vi "myRIO testing.vi"() -> (0 "Accelerometer":cluster{"Z":i16, "Y":i16, "X":i16} {"X" scale=-300.0..300.0; "Y" scale=-300.0..300.0; "Z" scale=-300.0..300.0})   [LabVIEW 2015, in "Everything.lvlib"]
uses:
  Everything.lvlib
  <vilib>/userdefined/High Color/IMAQdx.ctl
  <vilib>/myRIO/Common/Instrument Driver Framework/myRIO v1.0/UART/vis/myRIO v1.0 Close UART.vi
  <vilib>/FPGAPlugInAG/myRIO-1900/niLvFpga_Open_myRIO-1900.vi
  <vilib>/rvi/interface/common/dynamic/niFpgaDynamicAddResources.vi
  <vilib>/FPGAPlugInAG/Dynamic/niLvFpga_Run_Dynamic.vi
  <vilib>/Utility/error.llb/Error Cluster From Error Code.vi
  <vilib>/rvi/errors/niLvFpgaAdjustHostInterfaceError.vi
  <vilib>/FPGAPlugInAG/Dynamic/niLvFpga_Close_Dynamic.vi
  <vilib>/myRIO/Common/Instrument Driver Framework/Utilities/vis/FPGA Ref Manager.vi
  <vilib>/myRIO/Common/Instrument Driver Framework/myRIO v1.0/myRIO v1.0 Reset FPGA.vi
  <vilib>/myRIO/Common/Instrument Driver Framework/myRIO v1.0/IRQ/vis/myRIO v1.0 IRQ Info FGV.vi
  <vilib>/myRIO/Common/Instrument Driver Framework/myRIO v1.0/IRQ/vis/myRIO v1.0 Timer IRQ Info FGV.vi
  <vilib>/myRIO/Common/Instrument Driver Framework/myRIO v1.0/IRQ/vis/myRIO v1.0 ISR Agent.vi
  <vilib>/rvi/interface/nirviOpenFPGA/nirviOpenFPGA.xnode
  FPGA Bitfiles/PDMSMain_FPGATarget-Wi-Fi_Express2_Jo8xc+hAvHc.lvbitx
  FPGA/Express.vi
  <vilib>/rvi/interface/nirviMethod/nirviMethod.xnode
  <vilib>/rvi/interface/nirviReadWriteControl/nirviReadWriteControl.xnode
  <vilib>/rvi/interface/nirviCloseFPGA/nirviCloseFPGA.xnode
  <vilib>/myRIO/Instrument Drivers/Utilities/Utilities.lvlib
  NiFpgaLv.dll
  <vilib>/rvi/interface/Simulation/niFpgaSimulationCallBeginRW.vi
panel:
  in  "LED 0":T1 {"Brightness" max=1000}
  in  "LED 2":T2 {"Brightness" max=1000}
  in  "LED 1":T3 {"Brightness" max=1000}
  in  "LED 3":T4 {"Brightness" max=1000}
  out "IR":cluster{"1":bool, "2":bool}
  out "Image":T5(plugin-control)
  out "Error Out":errorcluster
  in  "Mot F":T6
  out "Button":bool
  out "PIR":bool
  in  "Stop Button":bool
  out "BOOL O/P":T7
  out "CM O/P":cluster{"US BK":u32, "US FL":u32, "US FR":u32}
  # "Obstacle"
  # "Robot's Position"
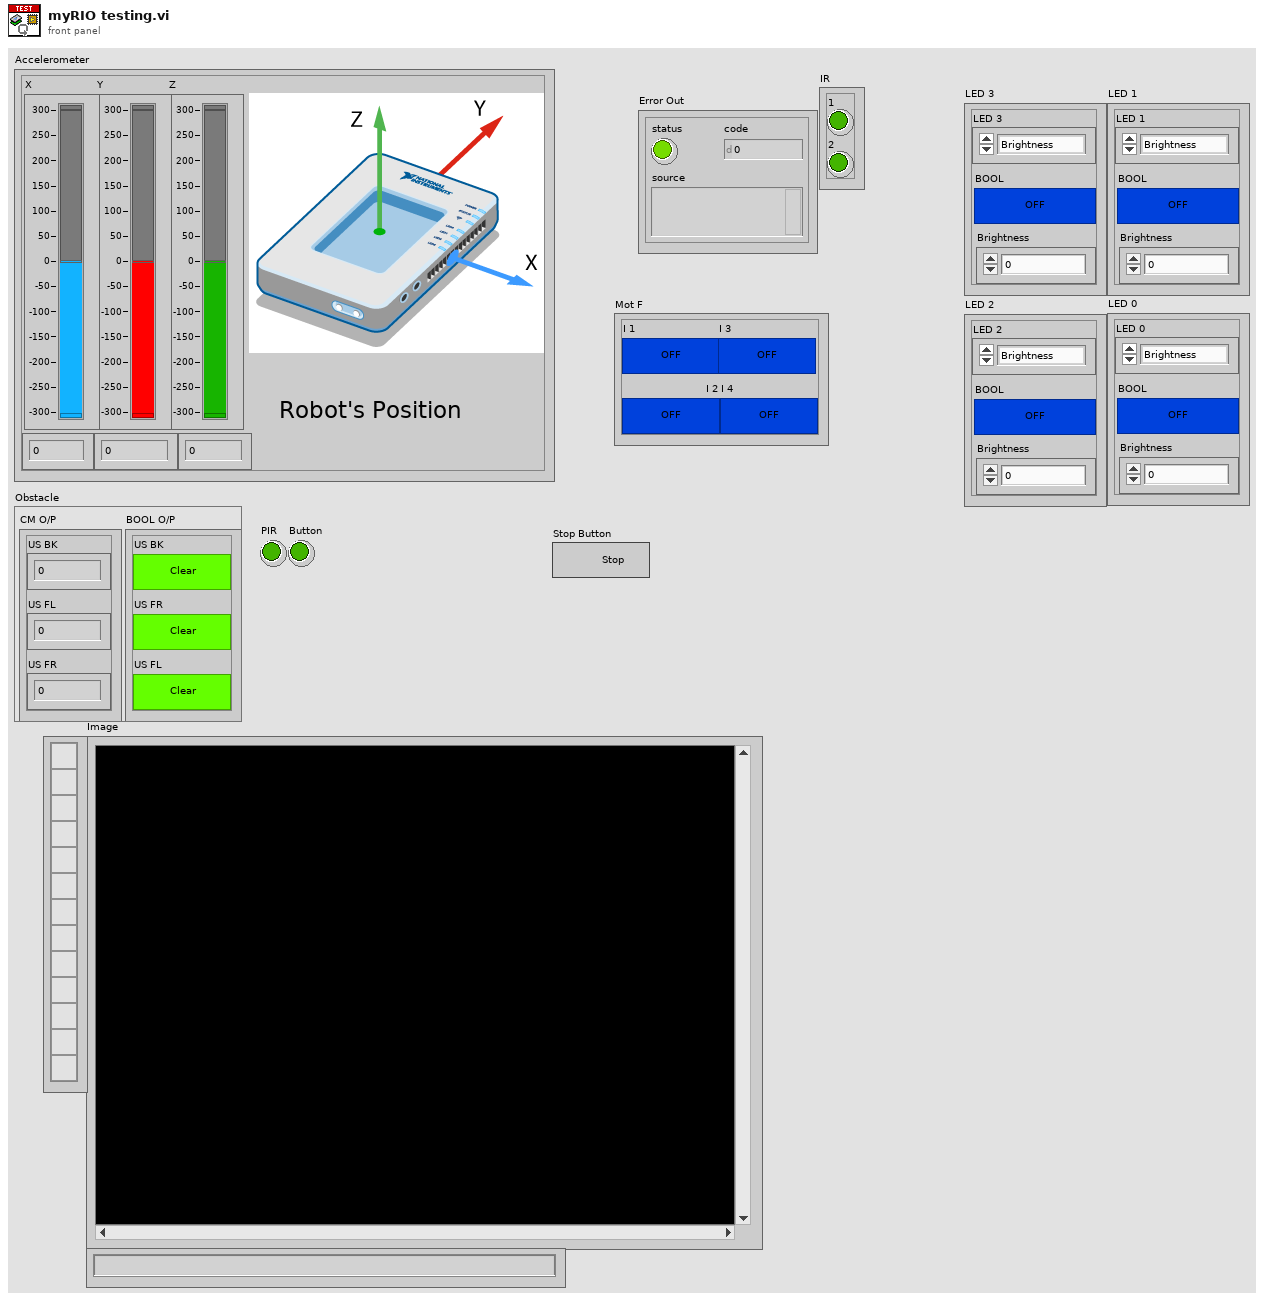
[diagram p1: front panel]
types:
  T1 = cluster{"LED 0":enum16{"Brightness", "Bool"}, "BOOL":bool, "Brightness":u32}
  T2 = cluster{"LED 2":enum16{"Brightness", "Bool"}, "BOOL":bool, "Brightness":u32}
  T3 = cluster{"LED 1":enum16{"Brightness", "Bool"}, "BOOL":bool, "Brightness":u32}
  T4 = cluster{"LED 3":enum16{"Brightness", "Bool"}, "BOOL":bool, "Brightness":u32}
  T5 = typedef "IMAQ Image.ctl" = refnum<image>
  T6 = cluster{"I 1":bool, "I 2":bool, "I 3":bool, "I 4":bool}
  T7 = cluster{"US BK":bool, "US FR":bool, "US FL":bool}
  T8 = typedef "IMAQdx.ctl" = refnum<k21>
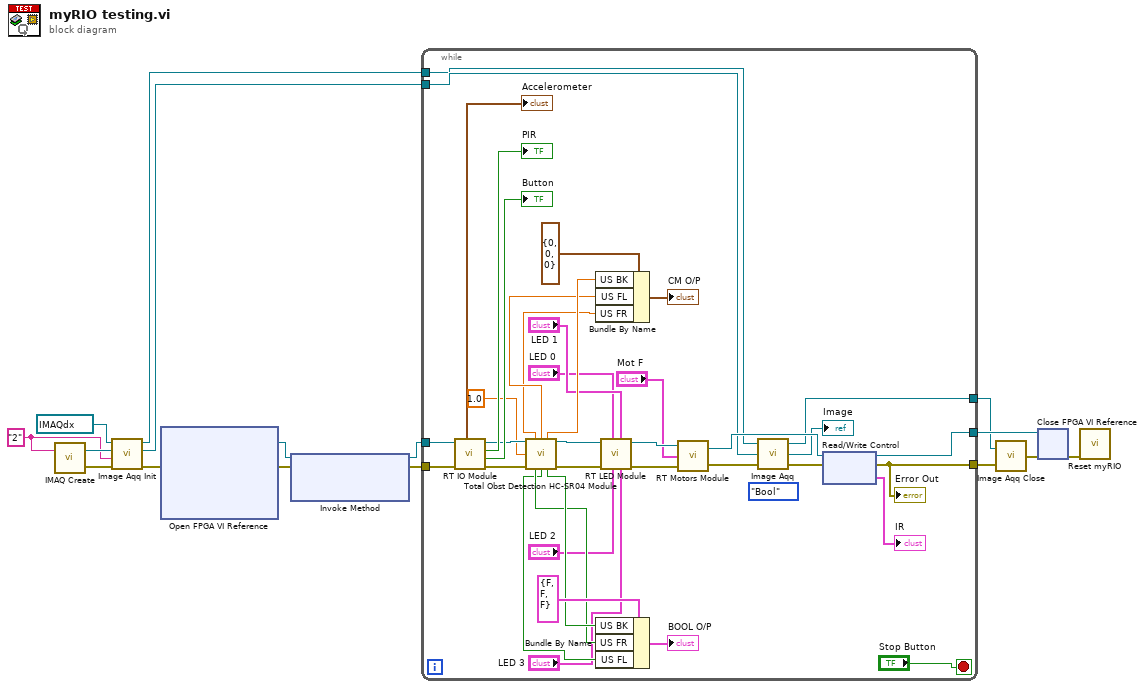
[diagram p0: block diagram]
diagram:
  w8 = "2" ("Image Name")
  n1 = call "IMAQ Create"("Image Name"=w8) -> ("New Image"=w14:T5, "error out"=w9:errorcluster)  [unwired: 4 in]
  n2 = call "Image Aqq Init.vi"("Error In"=w9, "Img Name In"=w8, "Img In"=w14, "Camera"=T8 "cam0") -> ("Error Out"=w7:errorcluster, "Img Out"=w12:T5, "Cam Out"=w11:T8)  [unwired: 1 out]
  n3 = xnode "Open FPGA VI Reference"("error in"=w7) -> ("FPGA VI Reference Out"=w4:refnum<k20>, "error out"=w3:errorcluster)  [unwired: 1 in]
  n4 = xnode "Invoke Method"("FPGA VI Reference In"=w4, "error in"=w3) -> ("FPGA VI Reference Out"=w2:refnum<k20>, "error out"=w1:errorcluster)  [unwired: 1 in]
  n5 = while {
    tunnel: w1 -> [w54]
    tunnel: [w34] -> w16
    tunnel: w2 -> [w32]
    tunnel: [w29] -> w13
    tunnel: w12 -> [w26]
    tunnel: w11 -> [w25]
    tunnel: [w24] -> w10
    stop <- "Stop Button" stop-if-true
    (unwired) enum16{"Brightness", "Bool"}."Bool" ("LED")
    n6 = call "RT IO Module.vi"("FPGA VI Reference In"=w32, "Error In"=w54) -> ("Accelerometer"=→"Accelerometer":cluster{"Z":i16, "Y":i16, "X":i16}, "FPGA VI Reference Out"=w31:refnum<k20>, "PIR"=→"PIR":bool, "Button"=→"Button":bool, "Error Out"=w51:errorcluster)  [unwired: 2 in, 2 out]
    n7 = call "Total Obst Detection HC-SR04 Module.vi"("FPGA VI Reference In"=w31, "Threshold"=sgl 1.0, "Error In"=w51) -> (1:"US FR"=w44:sgl, 2:"US FL"=w45:sgl, 3:"US BK"=w46:sgl, "FPGA VI Reference Out"=w39:refnum<k20>, 12:"US FR"=w42:bool, 13:"US FL"=w41:bool, 14:"US BK"=w43:bool, "Error Out"=w40:errorcluster)  [unwired: 5 in]
    n8 = Bundle By Name(cluster=cluster{"US BK":u32, "US FL":u32, "US FR":u32} {"US BK"=0, "US FL"=0, "US FR"=0} ("CM O/P 2"), "US BK"=w46, "US FL"=w45, "US FR"=w44) -> (→"CM O/P":cluster{"US BK":u32, "US FL":u32, "US FR":u32})
    n9 = Bundle By Name(cluster=T7 {"US BK"=FALSE, "US FR"=FALSE, "US FL"=FALSE} ("BOOL O/P 2"), "US BK"=w43, "US FR"=w42, "US FL"=w41) -> (→"BOOL O/P":T7)
    n10 = call "RT LED Module.vi"("LED 3"="LED 3", "LED 1"="LED 1", "LED 2"="LED 2", "LED 0"="LED 0", "error in"=w40, "FPGA VI Reference In"=w39) -> ("error out"=w38:errorcluster, "FPGA VI Reference Out"=w37:refnum<k20>)  [unwired: 4 in]
    n11 = call "RT Motors Module.vi"("Error In"=w38, "All"="Mot F", "FPGA VI Reference In"=w37) -> ("Error Out"=w27:errorcluster, "FPGA VI Reference Out"=w30:refnum<k20>)
    n12 = call "Image Aqq.vi"("Error In"=w27, "Img In"=w26, "Session In"=w25) -> ("Error Out"=w28:errorcluster, "Image"=→"Image":T5, "Cam Out"=w24:T8)
    n13 = xnode "Read/Write Control"("FPGA VI Reference In"=w30, "error in"=w28) -> ("FPGA VI Reference Out"=w34:refnum<k20>, "error out"=w29:errorcluster, "IR"=→"IR":cluster{"1":bool, "2":bool})
    "Error Out" <- w29
  }
  n14 = call "Image Aqq Close.vi"("Error In"=w13, "Session In"=w10) -> ("Error Out"=w5:errorcluster)
  n15 = xnode "Close FPGA VI Reference"("FPGA VI Reference In"=w16, "error in"=w5) -> ("error out"=w15:errorcluster)
  n16 = call <vilib>:"Reset myRIO.vi"("error in (no error)"=w15) -> ()  [unwired: 10 in, 1 out]
